vi "Test Backpressure.vi"() -> ()   [LabVIEW 2021]
uses:
  CIFChannels/Typedef/Direction.ctl
  ChannelCommon/typedef/FIFO Config.ctl
  ChannelCommon/typedef/TimeStamps.ctl
  CIF_CIPC_Fifo_U8.lvclass
  D:/dev/Packages/CIF_Channels_Core/src/CIPC_Channels/CIF_CIPC_Chan/CIF_CIPC_Chn.lvclass
  CIF_CIPC_Chan/CIF_CIPC_Chn.lvclass/CIF_CIPC_Chn.ctl
  CIF_CIPC_Chan/Accessors/Read Buffer Configuration.vi
  <vilib>/CIF Foundation/CIF Utilities/DataTypes/Flatten Unflatten/Flatten U64.vi
  <vilib>/CIF Foundation/CIF Utilities/DataTypes/Flatten Unflatten/Flatten U32.vi
  <vilib>/CIF Foundation/CIF Utilities/DataTypes/Flatten Unflatten/Flatten I32.vi
  ChannelCommon/ChannelCommon.lvlib
  CIFChannels/CIFChannels.lvclass
  CIF_CIPC_Chan/CIF_CIPC_Chn.lvclass
panel:
  out "status":string
  out "pass":bool
  out "error out":errorcluster
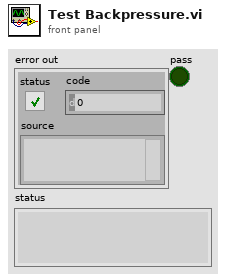
[diagram p1: front panel]
types:
  T1 = typedef "CIFChannels.lvclass/Direction.ctl" = enum16{"Publisher", "Subscriber"}
  T2 = typedef "ChannelCommon.lvlib/TimeStamps.ctl" = cluster{"ClockID":u8, "T0":i64, "T_Out":i64}
  T3 = typedef "ChannelCommon.lvlib/FIFO Config.ctl" = cluster{"Max Bytes/Msg":u64, "Max Msg/FIFO":u64, "Flags":u64}
  T4 = typedef "CIF_CIPC_Chn.lvclass/Buffer Configuration Data.ctl" = cluster{"Total Size":u32, "Read Size":u32, "Read Offset":u32, "CIPC BP References":T5, "Override CIPC Name":string, "Encoder Data":string}
  T5 = typedef "CIF_NI_CIPC.lvlib/Backpressure References.ctl" = cluster{"CIPC Reference":u64, "CIPC BP Reference":u64}
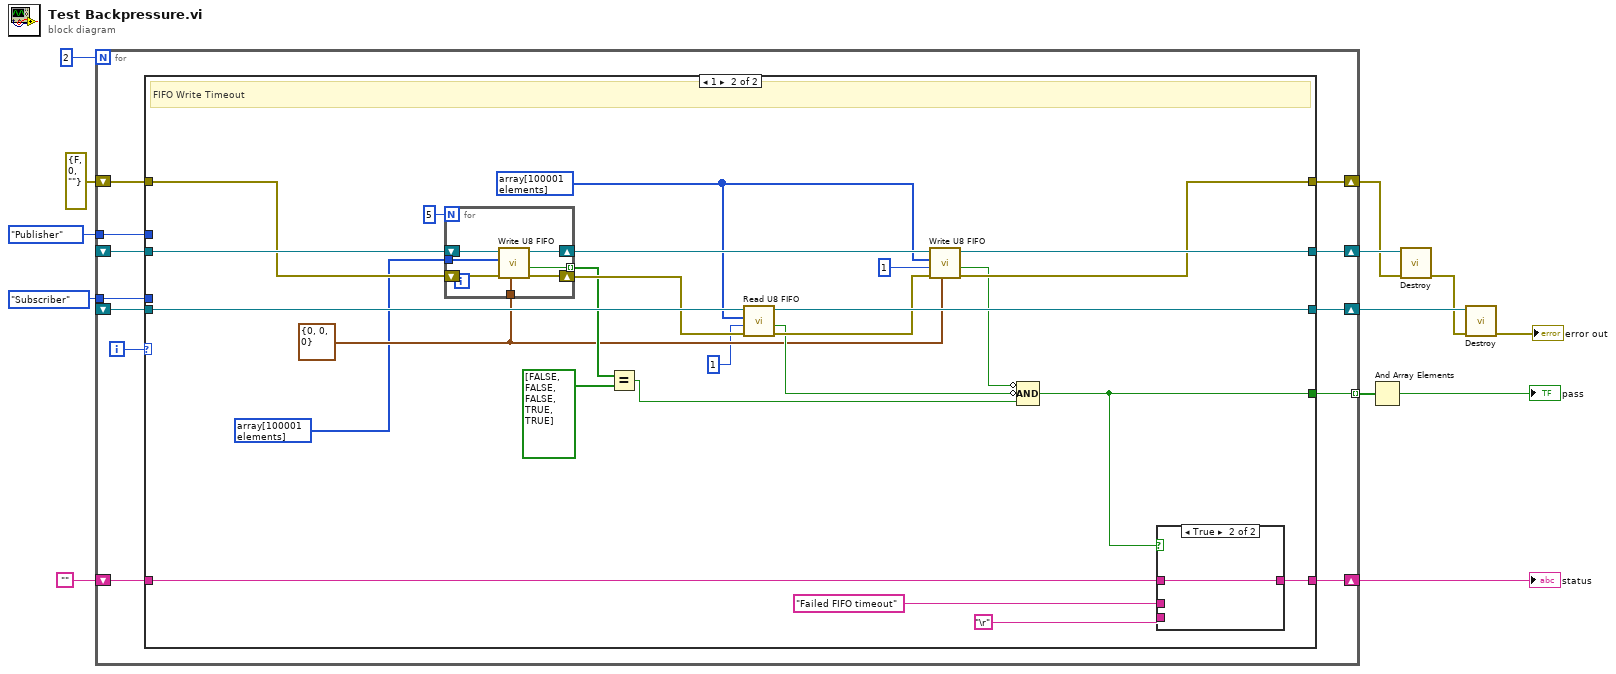
[diagram p0: block diagram]
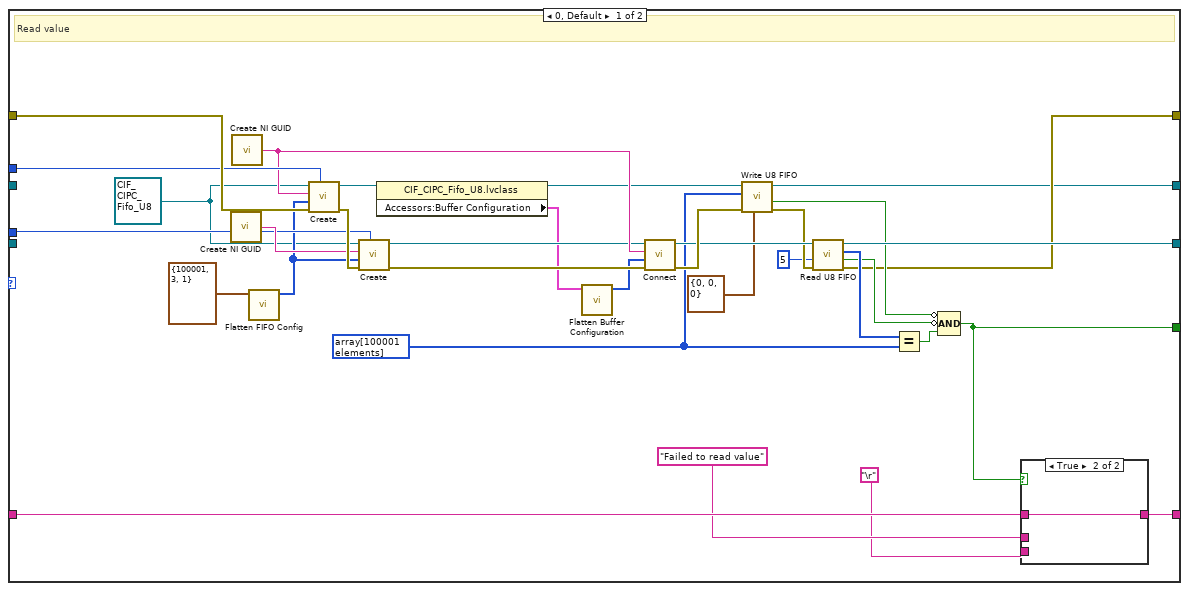
[diagram p2: hidden frame]
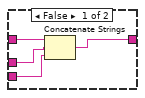
[diagram p3: hidden frame]
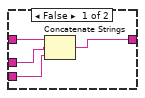
[diagram p4: hidden frame]
diagram:
  n1 = for {
    N: 2 -> [_]
    tunnel: [w25] -> w13 mode=indexing
    shift-right: [w23] -> w4
    shift-left: errorcluster {"status"=FALSE, "code"=0, "source"=""} ("error out") -> [w24]
    shift-right: [w20] -> w9
    shift-left: "" -> [w21]
    tunnel: Direction."Subscriber" ("Direction") -> [w19]
    tunnel: Direction."Publisher" ("Direction") -> [w18]
    shift-right: [w17] -> w3
    shift-left: _ -> [w15]
    shift-right: [w16] -> w5
    shift-left: _ -> [w14]
    i -> [w22]
    n2 = case shown="1" w22 {
      tunnel: [w53 w69] -> w25
      tunnel: w24 -> [w51 w83]
      tunnel: [w27 w75] -> w23
      tunnel: w21 -> [w58 w88]
      tunnel: [w57 w87] -> w20
      tunnel: w19 -> [w49 _]
      tunnel: w18 -> [w48 _]
      tunnel: [w41 w80] -> w17
      tunnel: [w26 w78] -> w16
      tunnel: w14 -> [_ w84]
      tunnel: w15 -> [_ w81]
      frame 0, Default {
        w35 = refnum<class "CIF_CIPC_Fifo_U8.lvclass"> refnum ("CIF_CIPC_Fifo_U8.lvclass")
        w29 = u8[] array[100001 elements] ("U8 Data")
        # "Read value"
        n3 = call <vilib>:"Create NI GUID.vi"() -> ("NI GUID"=w50:string)
        n4 = call <vilib>:"Create NI GUID.vi"() -> ("NI GUID"=w46:string)
        n5 = call "Flatten FIFO Config.vi"("FIFO Config in"=T3 {"Max Bytes/Msg"=100001, "Max Msg/FIFO"=3, "Flags"=1}) -> ("Flattened FIFO Config"=w36:u8[])  [unwired: 10 in]
        n6 = call-dynamic "Create.vi"("Direction"=w48, "error in (no error)"=w51, "Custom Config Data"=w36, "Name"=w46, "CIFFIFO in"=w35) -> ("error out"=w52:errorcluster, "CIFFIFO out"=w33:refnum<class "CIF_CIPC_Fifo_U8.lvclass">)  [unwired: 5 in]
        n7 = call-dynamic "Create.vi"("Direction"=w49, "error in (no error)"=w52, "Custom Config Data"=w36, "Name"=w50, "CIFFIFO in"=w35) -> ("error out"=w45:errorcluster, "CIFFIFO out"=w44:refnum<class "CIF_CIPC_Fifo_U8.lvclass">)  [unwired: 5 in]
        n8 = property class="CIF_CIPC_Fifo_U8.lvclass"(reference=w33) -> (reference out=w31:refnum<class "CIF_CIPC_Fifo_U8.lvclass">, "Accessors:Buffer Configuration"=w28:T4)  [unwired: 1 in, 1 out]
        n9 = call "Flatten Buffer Configuration.vi"("Buffer Configuration"=w28) -> ("Flattened Configuration"=w32:u8[])  [unwired: 10 in]
        n10 = call-dynamic "Connect.vi"("error in (no error)"=w45, "Custom Config Data"=w32, "Connection Name"=w46, "CIFTag in"=w44) -> ("error out"=w43:errorcluster, "CIFTag out"=w42:refnum<class "CIF_CIPC_Fifo_U8.lvclass">)  [unwired: 6 in]
        n11 = call-dynamic "Write U8 FIFO.vi"("FIFO Timestamps"=T2 {"ClockID"=0, "T0"=0, "T_Out"=0}, "error in (no error)"=w43, "Data in"=w29, "CIFFIFO in"=w31) -> ("error out"=w40:errorcluster, "timed out?"=w39:bool, "CIFFIFO out"=w26:refnum<class "CIF_CIPC_Fifo_U8.lvclass">)  [unwired: 4 in, 1 out]
        n12 = call-dynamic "Read U8 FIFO.vi"("error in (no error)"=w40, "Timeout (ms)"=5, "CIFFIFO in"=w42) -> ("error out"=w27:errorcluster, "timed out?"=w37:bool, "Data out"=w38:u8[], "CIFFIFO out"=w41:refnum<class "CIF_CIPC_Fifo_U8.lvclass">)  [unwired: 4 in, 1 out]
        n13 = Equal?(x=w38, y=w29) -> (x = y?=w54:bool)
        n14 = Compound Arithmetic op=AND(invert w39, invert w37, w54) -> (w53:bool)
        n15 = case shown="True" w53 {
          tunnel: w58 -> [w62 w63]
          tunnel: [w59 w63] -> w57
          tunnel: "Failed to read value" -> [w61 _]
          tunnel: "\r" -> [w60 _]
          frame False {
            n16 = Concatenate Strings(w62, w61, w60) -> (w59:string)
          }
          frame True {
          }
        }
      }
      frame 1 {
        w66 = u8[] array[100001 elements] ("U8 Data")
        w68 = T2 {"ClockID"=0, "T0"=0, "T_Out"=0} ("FIFO Timestamps")
        # "FIFO Write Timeout"
        n17 = for {
          N: 5 -> [_]
          tunnel: u8[] array[100001 elements] ("U8 Data") -> [w93]
          tunnel: w68 -> [w92]
          shift-right: [w91] -> w79
          shift-left: w84 -> [w95]
          tunnel: [w90] -> w74 mode=indexing
          shift-right: [w89] -> w77
          shift-left: w83 -> [w94]
          n18 = call-dynamic "Write U8 FIFO.vi"("FIFO Timestamps"=w92, "error in (no error)"=w94, "Data in"=w93, "CIFFIFO in"=w95) -> ("error out"=w89:errorcluster, "timed out?"=w90:bool, "CIFFIFO out"=w91:refnum<class "CIF_CIPC_Fifo_U8.lvclass">)  [unwired: 4 in, 1 out]
        }
        n19 = Equal?(x=w74, y=bool[] [FALSE, FALSE, FALSE, TRUE, TRUE]) -> (x = y?=w70:bool)
        n20 = call-dynamic "Read U8 FIFO.vi"("error in (no error)"=w77, "Timeout (ms)"=1, "Data in"=w66, "CIFFIFO in"=w81) -> ("error out"=w76:errorcluster, "timed out?"=w72:bool, "CIFFIFO out"=w80:refnum<class "CIF_CIPC_Fifo_U8.lvclass">)  [unwired: 3 in, 2 out]
        n21 = call-dynamic "Write U8 FIFO.vi"("FIFO Timestamps"=w68, "error in (no error)"=w76, "Timeout (ms)"=1, "Data in"=w66, "CIFFIFO in"=w79) -> ("error out"=w75:errorcluster, "timed out?"=w71:bool, "CIFFIFO out"=w78:refnum<class "CIF_CIPC_Fifo_U8.lvclass">)  [unwired: 3 in, 1 out]
        n22 = Compound Arithmetic op=AND(invert w71, invert w72, w70) -> (w69:bool)
        n23 = case shown="True" w69 {
          tunnel: w88 -> [w99 w100]
          tunnel: [w96 w100] -> w87
          tunnel: "Failed FIFO timeout" -> [w98 _]
          tunnel: "\r" -> [w97 _]
          frame False {
            n24 = Concatenate Strings(w99, w98, w97) -> (w96:string)
          }
          frame True {
          }
        }
      }
    }
  }
  "status" <- w9
  n25 = And Array Elements(Boolean array=w13) -> (logical AND=→"pass":bool)
  n26 = call-dynamic "Destroy.vi"("error in (no error)"=w4, "CIFTag in"=w5) -> ("error out"=w2:errorcluster)  [unwired: 8 in, 1 out]
  n27 = call-dynamic "Destroy.vi"("error in (no error)"=w2, "CIFTag in"=w3) -> ("error out"=→"error out":errorcluster)  [unwired: 8 in, 1 out]
